vi "IDrawable Draw.vi"(7 "Drawing Settings":T1, 8 "error in (no error)":errorcluster, 10 "2D Picture":picture, 11 "Food in":refnum<class "Food.lvclass">) -> (0 "error out":errorcluster, 2 "2D Picture out":picture, 3 "Food out":refnum<class "Food.lvclass">)   [LabVIEW 2020, in "Food.lvclass"]
uses:
  Food.lvclass
  Drawing Settings STYP.ctl
  Food.lvclass/Food.ctl
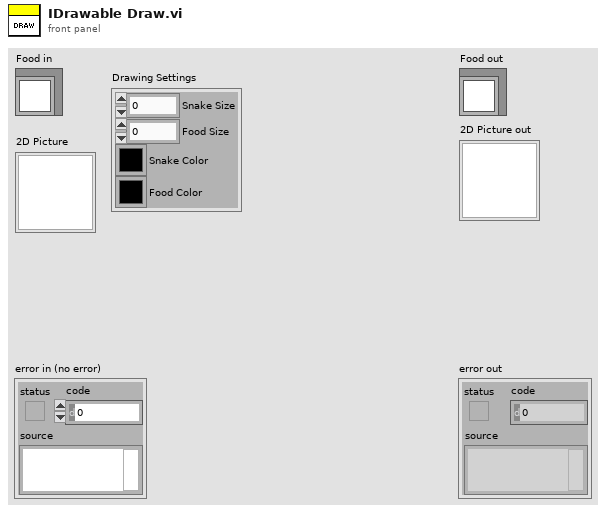
[diagram p1: front panel]
types:
  T1 = typedef "Drawing Settings STYP.ctl" = cluster{"Snake Size":u32, "Food Size":u32, "Snake Color":u32, "Food Color":u32}
  T2 = cluster{"left":i16, "top":i16, "right":i16, "bottom":i16}
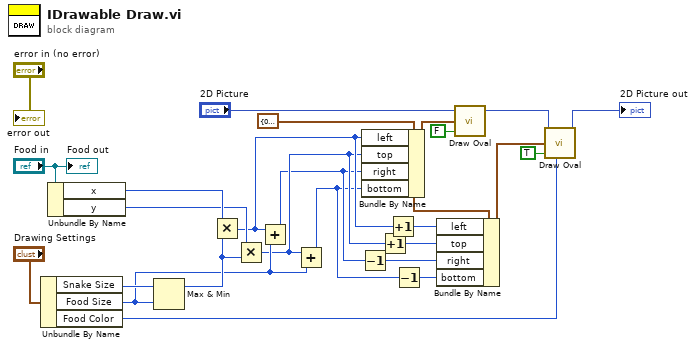
[diagram p0: block diagram]
diagram:
  w10 = T2 {"left"=0, "top"=0, "right"=0, "bottom"=0} ("rect")
  n1 = Unbundle By Name("Drawing Settings") -> ("Snake Size"=w23:u32, "Food Size"=w19:u32, "Food Color"=w13:u32)
  n2 = Unbundle By Name("Food in") -> ("x"=w22:u32, "y"=w21:u32)
  n3 = Max & Min(x=w23, y=w19) -> (max(x,y)=w20:u32)  [unwired: 1 out]
  n4 = Multiply(x=w22, y=w20) -> (x*y=w8:u32)
  n5 = Multiply(x=w21, y=w20) -> (x*y=w7:u32)
  n6 = Add(x=w8, y=w19) -> (x+y=w6:u32)
  n7 = Add(x=w7, y=w19) -> (x+y=w5:u32)
  n8 = Decrement(x=w6) -> (x-1=w2:u32)
  n9 = Bundle By Name(cluster=w10, "left"=w8, "top"=w7, "right"=w6, "bottom"=w5) -> (w11:T2)
  n10 = Increment(x=w7) -> (x+1=w3:u32)
  n11 = Increment(x=w8) -> (x+1=w4:u32)
  n12 = Decrement(x=w5) -> (x-1=w1:u32)
  n13 = Bundle By Name(cluster=w10, "left"=w4, "top"=w3, "right"=w2, "bottom"=w1) -> (w9:T2)
  n14 = call <vilib>:"Draw Oval.vi"("picture"="2D Picture", "rect"=w11, "fill?(F)"=FALSE) -> ("new picture"=w15:picture)  [unwired: 6 in]
  n15 = call <vilib>:"Draw Oval.vi"("picture"=w15, "rect"=w9, "fill?(F)"=TRUE, "color(black)"=w13) -> ("new picture"=→"2D Picture out":picture)  [unwired: 5 in]
  "error out" <- "error in (no error)"
  "Food out" <- "Food in"
